vi "Display and Select Steps.vi"(4 "Sequence Context":T1) -> (0 "error out":errorcluster, 1 "Test Data":T2 {"Numeric Measurement" format="%.2f"})   [LabVIEW 2013]
uses:
  Demo/LabVIEW/SupportVIs.llb/LabVIEW Test - Test Data.ctl
  <vilib>/addons/TestStand/_TSLegacy.llb/LabVIEW Test - Sequence Context.ctl
panel:
  in  "Main Sequence":i32[](listbox)
  in  "done":bool
  # "(Shift-Click to select steps)"
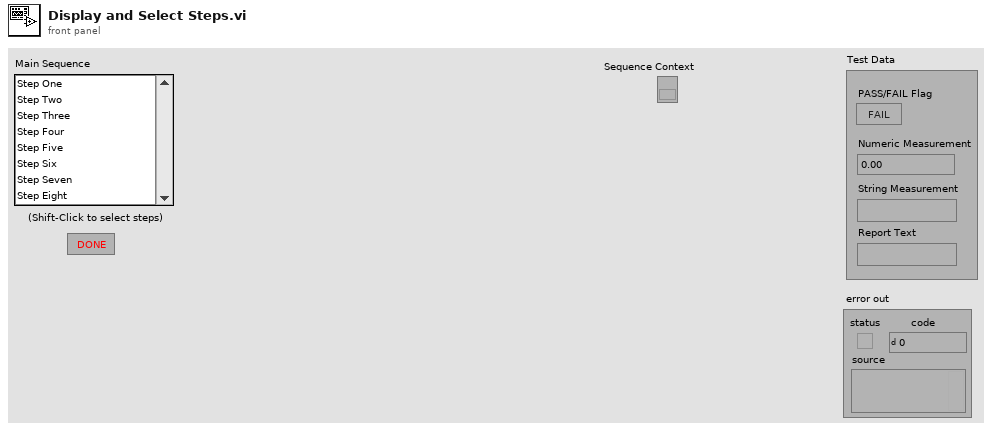
[diagram p1: front panel]
types:
  T1 = typedef "LabVIEW Test - Sequence Context.ctl" = refnum<k7>
  T2 = typedef "LabVIEW Test - Test Data.ctl" = cluster{"PASS/FAIL Flag":bool, "Numeric Measurement":dbl, "String Measurement":string, "Report Text":string}
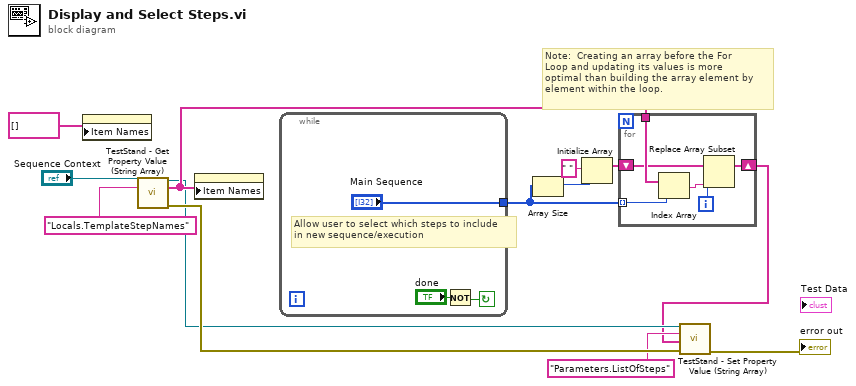
[diagram p0: block diagram]
diagram:
  # "Note:  Creating an array before the For \nLoop and updating its values is more \noptimal than building the array element by \nelement within the loop."
  n1 = property on="Main Sequence" class="LstBox (strict)"("Item Names"=string[] [] ("Array Constant")) -> ()  [unwired: 2 in, 2 out]
  n2 = call <vilib>:"TestStand - Get Property Value (String Array).vi"("Sequence Context In"="Sequence Context", "Lookup String"="Locals.TemplateStepNames") -> ("Sequence Context Out"=w9:refnum<k7>, "Value"=w11:string[], "error out"=w10:errorcluster)  [unwired: 1 in, 10 out]
  n3 = property on="Main Sequence" class="LstBox (strict)"("Item Names"=w11) -> ()  [unwired: 2 in, 2 out]
  n4 = while {
    tunnel: ["Main Sequence"] -> w2
    stop <- w14 continue-if-true
    # "Allow user to select which steps to include\nin new sequence/execution"
    n5 = Not(x="done") -> (.not. x?=w14:bool)
  }
  n6 = Array Size(array=w2) -> (size(s)=w1:i32)
  n7 = Initialize Array(" ", w1) -> (w6:string[])
  n8 = for {
    tunnel: w2 -> [w21] mode=indexing
    tunnel: w11 -> [w22]
    shift-right: [w18] -> w7
    shift-left: w6 -> [w20]
    i -> [w19]
    n9 = Index Array(array=w22, index=w21) -> (element=w17:string)
    n10 = Replace Array Subset(array=w20, new element=w17, index=w19) -> (w18:string[])
  }
  n11 = call <vilib>:"TestStand - Set Property Value (String Array).vi"("Sequence Context In"=w9, "Lookup String"="Parameters.ListOfSteps", "New Value"=w7, "error in (no error)"=w10) -> ("error out"=→"error out":errorcluster)  [unwired: 1 in, 10 out]
